vi "Create Tree.vi"(7 "Tree Refnum":refnum<vi>, 8 "error in":errorcluster, 9 "Parent Tag":string, 10 "palette data 2":T5={"display name"="", "view format"=0, "palette width"=4, "items"=[], "256 color icon"=bytes[0], "B&W color icon"=bytes[0], "help information"={"help tag"="", "help file path"=path ""}, "palette description"="", "synchronize information"={"synchronize with directory"=FALSE, "synchronize directory path"=path ""}} {"view format" items=["Icons", "Text", "Icons and Text"]}, 11 "palette data 1":T5={"display name"="", "view format"=0, "palette width"=4, "items"=[], "256 color icon"=bytes[0], "B&W color icon"=bytes[0], "help information"={"help tag"="", "help file path"=path ""}, "palette description"="", "synchronize information"={"synchronize with directory"=FALSE, "synchronize directory path"=path ""}} {"view format" items=["Icons", "Text", "Icons and Text"]}) -> (0 "error out":errorcluster, 2 "data array 2":cluster{"Label":string, "Data":variant}[](array[cluster]), 3 "data array 1":cluster{"Label":string, "Data":variant}[](array[cluster]))   [LabVIEW 2017]
uses:
  <vilib>/Palette API/Palette Menu/Public Type Define/View Format.ctl
  <vilib>/Palette API/Palette Menu/Public Type Define/Items.ctl
  <vilib>/Palette API/Palette Menu/Public Type Define/Item.ctl
  <vilib>/Palette API/Palette Menu/Public Type Define/Synchronize Info.ctl
  <vilib>/Palette API/Palette Menu/Palette Menu.lvlib
panel:
  in  "array size 1":i32
  in  "array size 2":i32
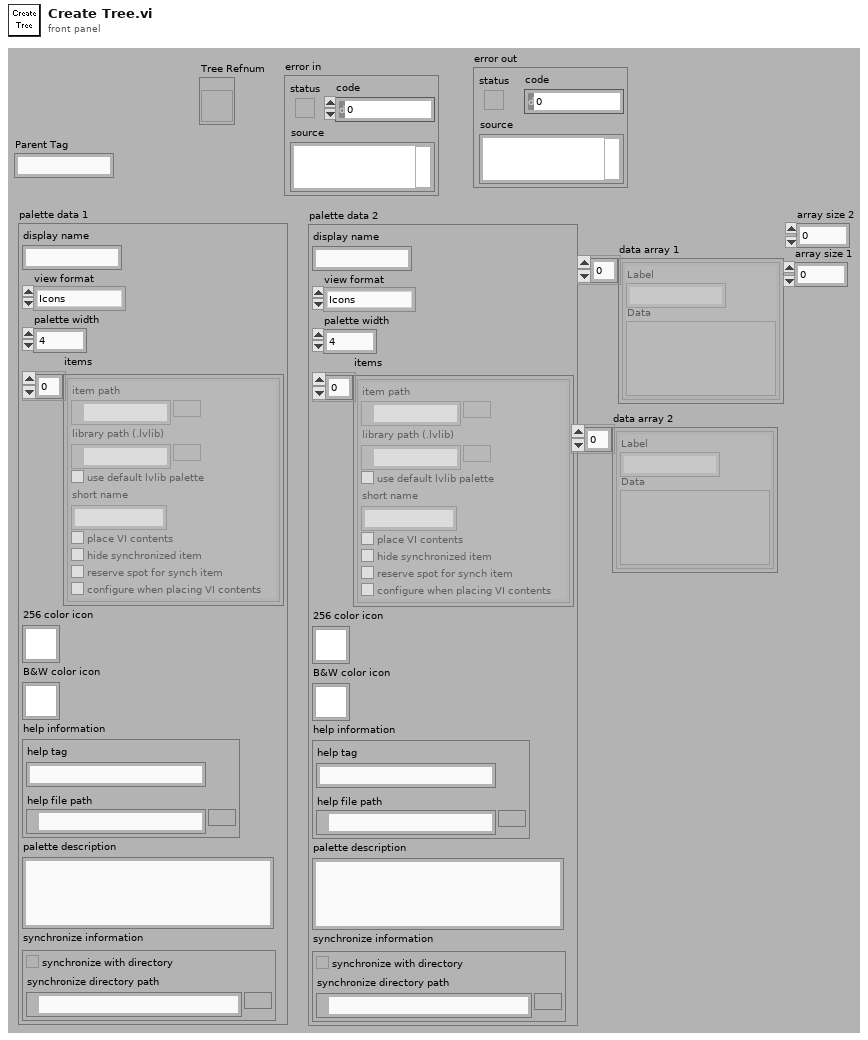
[diagram p1: front panel]
types:
  T1 = typedef "Palette Menu.lvlib/View Format.ctl" = u16
  T2 = typedef "Palette Menu.lvlib/Items.ctl" = T3[]
  T3 = typedef "Palette Menu.lvlib/Item.ctl" = cluster{"item path":path, "library path (.lvlib)":path, "use default lvlib palette":bool, "short name":string, "place VI contents":bool, "hide synchronized item":bool, "reserve spot for synch item":bool, "configure when placing VI contents":bool}
  T4 = typedef "Palette Menu.lvlib/Synchronize Info.ctl" = cluster{"synchronize with directory":bool, "synchronize directory path":path}
  T5 = cluster{"display name":string, "view format":T1, "palette width":i16, "items":T2, "256 color icon":picture, "B&W color icon":picture, "help information":cluster{"help tag":string, "help file path":path}, "palette description":string, "synchronize information":T4}
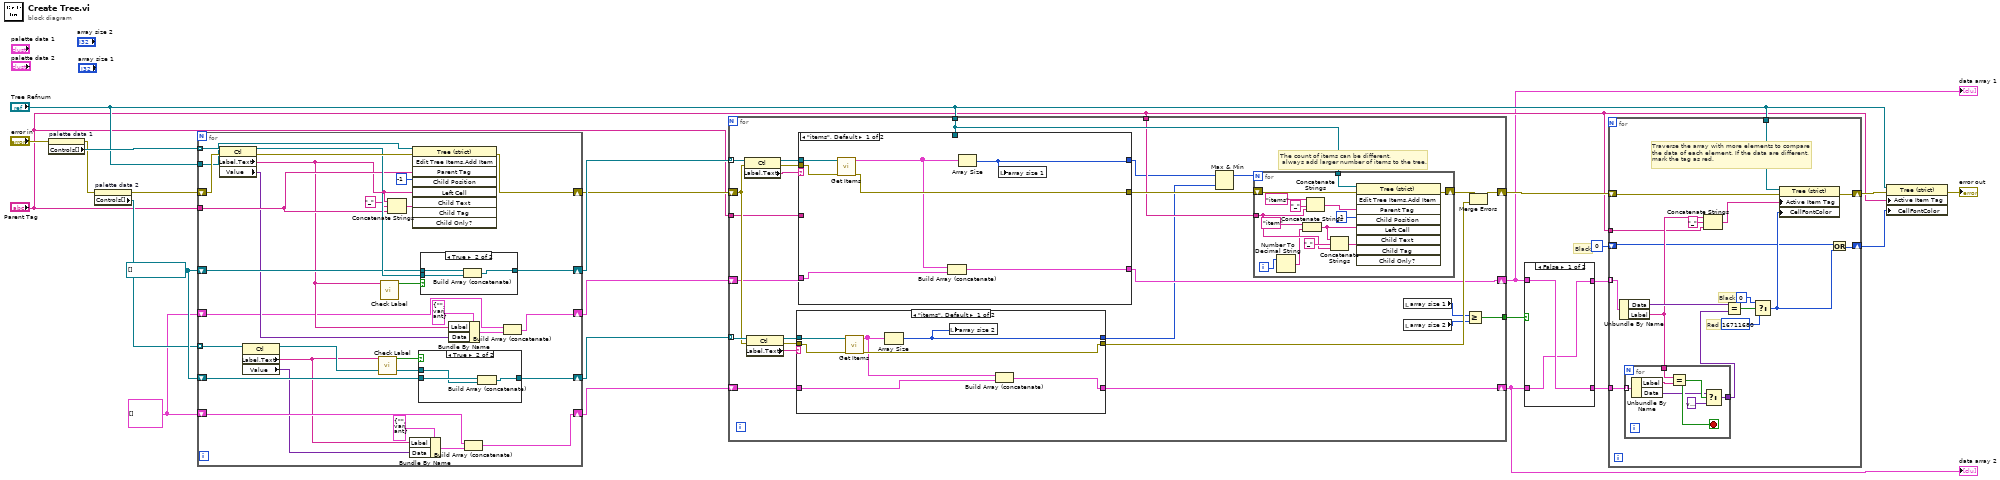
[diagram p0: block diagram]
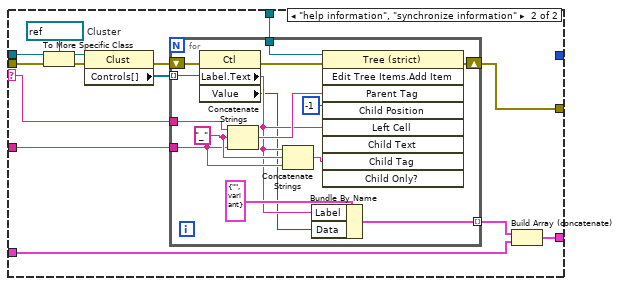
[diagram p3: hidden frame]
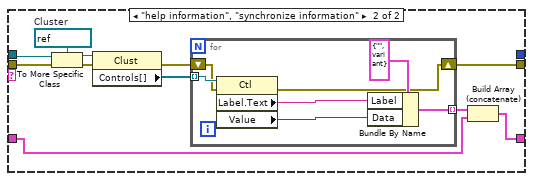
[diagram p4: hidden frame]
diagram:
  w16 = cluster{"Label":string, "Data":variant}[] []
  w24 = refnum<vi>[] []
  # "Black"
  n1 = property on="palette data 1" class="Clust (strict)"(error in="error in") -> (error out=w19:errorcluster, "Controls[]"=w21:refnum<vi>[])  [unwired: 1 in, 1 out]
  n2 = property on="palette data 2" class="Clust (strict)"(error in=w19) -> (error out=w18:errorcluster, "Controls[]"=w17:refnum<vi>[])  [unwired: 1 in, 1 out]
  n3 = for {
    tunnel: w21 -> [w53] mode=indexing
    shift-right: [w50] -> w22
    shift-left: w24 -> [w46]
    shift-right: [w37] -> w12
    shift-left: w18 -> [w49]
    tunnel: "Parent Tag" -> [w39]
    tunnel: w17 -> [w48] mode=indexing
    shift-right: [w45] -> w23
    shift-left: w24 -> [w44]
    tunnel: "Tree Refnum" -> [w43]
    shift-right: [w25] -> w15
    shift-left: w16 -> [w28]
    shift-right: [w31] -> w14
    shift-left: w16 -> [w32]
    n4 = property class="Ctl"(reference=w53, error in=w49) -> (reference out=w51:refnum<vi>, error out=w54:errorcluster, "Label.Text"=w33:string, "Value"=w34:variant)
    n5 = property class="Ctl"(reference=w48) -> (reference out=w47:refnum<vi>, "Label.Text"=w26:string, "Value"=w27:variant)  [unwired: 1 in, 1 out]
    n6 = call "Check Label.vi"("Label"=w26) -> ("Boolean"=w38:bool)  [unwired: 10 out]
    n7 = call "Check Label.vi"("Label"=w33) -> ("Boolean"=w52:bool)  [unwired: 10 out]
    n8 = Concatenate Strings(w33, "_" ("string"), w39) -> (w40:string)
    n9 = Bundle By Name(cluster=cluster{"Label":string, "Data":variant} {"Label"="", "Data"=variant} ("data cluster"), "Label"=w26, "Data"=w27) -> (w29:cluster{"Label":string, "Data":variant})
    n10 = invoke on="Invoke Node" class="Tree (strict)" method="Edit Tree Items.Add Item"(reference=w43, error in=w54, "Parent Tag"=w39, "Child Position"=-1, "Left Cell"=w33, "Child Tag"=w40) -> (error out=w37:errorcluster)  [unwired: 3 in, 8 out]
    n11 = case shown="True" w38 {
      tunnel: w47 -> [_ w56]
      tunnel: [w55 w58] -> w45
      tunnel: w44 -> [w55 w57]
      frame False {
      }
      frame True {
        n12 = Build Array (concatenate)(w57, w56) -> (w58:refnum<vi>[])
      }
    }
    n13 = case shown="True" w52 {
      tunnel: w51 -> [_ w60]
      tunnel: [w59 w62] -> w50
      tunnel: w46 -> [w59 w61]
      frame False {
      }
      frame True {
        n14 = Build Array (concatenate)(w61, w60) -> (w62:refnum<vi>[])
      }
    }
    n15 = Bundle By Name(cluster=cluster{"Label":string, "Data":variant} {"Label"="", "Data"=variant} ("data cluster"), "Label"=w33, "Data"=w34) -> (w35:cluster{"Label":string, "Data":variant})
    n16 = Build Array (concatenate)(w28, w29) -> (w25:cluster{"Label":string, "Data":variant}[])
    n17 = Build Array (concatenate)(w32, w35) -> (w31:cluster{"Label":string, "Data":variant}[])
  }
  n18 = for {
    tunnel: w22 -> [w88] mode=indexing
    shift-right: [w78] -> w13
    shift-left: w12 -> [w80]
    tunnel: w23 -> [w84] mode=indexing
    tunnel: "Tree Refnum" -> [w70]
    tunnel: "Parent Tag" -> [w77]
    shift-right: [w74] -> w1
    shift-left: w15 -> [w76]
    shift-right: [w73] -> w2
    shift-left: w14 -> [w75]
    tunnel: "Parent Tag" -> [w69]
    tunnel: [w67] -> w5
    # "The count of items can be different,\n always add larger number of items to the tree."
    n19 = property class="Ctl"(reference=w88, error in=w80) -> (reference out=w86:refnum<vi>, error out=w85:errorcluster, "Label.Text"=w87:string)
    n20 = property class="Ctl"(reference=w84, error in=w80) -> (reference out=w82:refnum<vi>, error out=w81:errorcluster, "Label.Text"=w83:string)
    n21 = case shown="\"items\", Default" w83 {
      tunnel: w82 -> [w145 w156]
      tunnel: w81 -> [w142 w155]
      tunnel: [w141 w146] -> w79
      tunnel: w76 -> [w144 w148]
      tunnel: [w143 w147] -> w74
      tunnel: [w139 _] -> w65
      frame "items", Default {
        n22 = call "Get Items.vi"("error in"=w142, "Ctl Refnum"=w145) -> ("error out"=w141:errorcluster, "items array"=w140:cluster{"Label":string, "Data":variant}[])  [unwired: 8 out]
        n23 = Array Size(array=w140) -> (size(s)=w139:i32)
        n24 = local write "array size 2"(w139) -> ()
        n25 = Build Array (concatenate)(w140, w144) -> (w143:cluster{"Label":string, "Data":variant}[])
      }
      frame "help information", "synchronize information" {
        w154 = refnum<vi> refnum  # Cluster
        n26 = To More Specific Class(target class=w154, reference=w156, error in=w155) -> (specific class reference=w152:refnum<vi>, error out=w153:errorcluster)
        n27 = property class="Clust"(reference=w152, error in=w153) -> (error out=w150:errorcluster, "Controls[]"=w151:refnum<vi>[])  [unwired: 1 out]
        n28 = for {
          tunnel: w151 -> [w163] mode=indexing
          shift-right: [w157] -> w146
          shift-left: w150 -> [w162]
          tunnel: [w158] -> w149 mode=indexing
          n29 = property class="Ctl"(reference=w163, error in=w162) -> (error out=w157:errorcluster, "Label.Text"=w160:string, "Value"=w159:variant)  [unwired: 1 out]
          n30 = Bundle By Name(cluster=cluster{"Label":string, "Data":variant} {"Label"="", "Data"=variant} ("data cluster"), "Label"=w160, "Data"=w159) -> (w158:cluster{"Label":string, "Data":variant})
        }
        n31 = Build Array (concatenate)(w149, w148) -> (w147:cluster{"Label":string, "Data":variant}[])
      }
    }
    n32 = case shown="\"items\", Default" w87 {
      selector: w87 -> [_ w118]
      tunnel: w86 -> [w109 w123]
      tunnel: w85 -> [w106 w122]
      tunnel: [w105 w116] -> w72
      tunnel: w77 -> [_ w114]
      tunnel: w75 -> [w108 w112]
      tunnel: [w107 w111] -> w73
      tunnel: w70 -> [_ w110]
      tunnel: [w103 _] -> w66
      frame "items", Default {
        n33 = call "Get Items.vi"("error in"=w106, "Ctl Refnum"=w109) -> ("error out"=w105:errorcluster, "items array"=w104:cluster{"Label":string, "Data":variant}[])  [unwired: 8 out]
        n34 = Build Array (concatenate)(w104, w108) -> (w107:cluster{"Label":string, "Data":variant}[])
        n35 = Array Size(array=w104) -> (size(s)=w103:i32)
        n36 = local write "array size 1"(w103) -> ()
      }
      frame "help information", "synchronize information" {
        w121 = refnum<vi> refnum  # Cluster
        n37 = To More Specific Class(target class=w121, reference=w123, error in=w122) -> (specific class reference=w119:refnum<vi>, error out=w120:errorcluster)
        n38 = property class="Clust"(reference=w119, error in=w120) -> (error out=w117:errorcluster, "Controls[]"=w115:refnum<vi>[])  [unwired: 1 out]
        n39 = for {
          tunnel: w115 -> [w138] mode=indexing
          tunnel: w118 -> [w132]
          shift-right: [w135] -> w116
          shift-left: w117 -> [w134]
          tunnel: w110 -> [w133]
          tunnel: w114 -> [w129]
          tunnel: [w124] -> w113 mode=indexing
          w130 = "_" ("string")
          n40 = property class="Ctl"(reference=w138, error in=w134) -> (error out=w137:errorcluster, "Label.Text"=w126:string, "Value"=w125:variant)  [unwired: 1 out]
          n41 = Concatenate Strings(w132, w130, w129) -> (w131:string)
          n42 = Concatenate Strings(w126, w130, w129) -> (w128:string)
          n43 = Bundle By Name(cluster=cluster{"Label":string, "Data":variant} {"Label"="", "Data"=variant} ("data cluster"), "Label"=w126, "Data"=w125) -> (w124:cluster{"Label":string, "Data":variant})
          n44 = invoke on="Invoke Node" class="Tree (strict)" method="Edit Tree Items.Add Item"(reference=w133, error in=w137, "Parent Tag"=w131, "Child Position"=-1, "Left Cell"=w126, "Child Tag"=w128) -> (error out=w135:errorcluster)  [unwired: 3 in, 8 out]
        }
        n45 = Build Array (concatenate)(w113, w112) -> (w111:cluster{"Label":string, "Data":variant}[])
      }
    }
    n46 = Max & Min(x=w66, y=w65) -> (max(x,y)=w68:i32)  [unwired: 1 out]
    n47 = for {
      N: w68 -> [_]
      tunnel: w70 -> [w101]
      shift-right: [w100] -> w71
      shift-left: w72 -> [w99]
      tunnel: w69 -> [w95]
      i -> [w90]
      n48 = Number To Decimal String(number=w90) -> (decimal integer string=w92:string)  [unwired: 1 out]
      n49 = Concatenate Strings("item" ("string"), w92) -> (w91:string)
      n50 = Concatenate Strings("items" ("Parent Tag"), "_" ("string"), w95) -> (w97:string)
      n51 = Concatenate Strings(w91, "_" ("string"), w95) -> (w94:string)
      n52 = invoke on="Invoke Node" class="Tree (strict)" method="Edit Tree Items.Add Item"(reference=w101, error in=w99, "Parent Tag"=w97, "Child Position"=-1, "Left Cell"=w91, "Child Tag"=w94) -> (error out=w100:errorcluster)  [unwired: 3 in, 8 out]
    }
    n53 = local read "array size 1"() -> (w64:i32)
    n54 = local read "array size 2"() -> (w63:i32)
    n55 = Greater Or Equal?(x=w64, y=w63) -> (x >= y?=w67:bool)
    n56 = Merge Errors(w71, w79) -> (w78:errorcluster)
  }
  "data array 1" <- w2
  "data array 2" <- w1
  n57 = case shown="False" w5 {
    tunnel: [w164 w167] -> w4
    tunnel: w2 -> [w165 w167]
    tunnel: w1 -> [w164 w166]
    tunnel: [w165 w166] -> w3
    frame False {
    }
    frame True {
    }
  }
  n58 = for {
    shift-right: [w176] -> w10
    shift-left: w13 -> [w177]
    tunnel: w4 -> [w184] mode=indexing
    tunnel: w3 -> [w171]
    tunnel: "Tree Refnum" -> [w178]
    tunnel: "Parent Tag" -> [w173]
    shift-right: [w169] -> w7
    shift-left: u32 0 -> [w168]
    # "Traverse the array with more elements to compare\nthe data of each element. If the data are different, \nmark the tag as red."
    # "Red"
    # "Black"
    n59 = Unbundle By Name(w184) -> ("Data"=w181:variant, "Label"=w175:string)
    n60 = for {
      tunnel: w171 -> [w191] mode=indexing
      tunnel: w175 -> [w189]
      tunnel: [w185] -> w180
      stop <- w188 stop-if-true
      n61 = Unbundle By Name(w191) -> ("Label"=w190:string, "Data"=w187:variant)
      n62 = Equal?(x=w189, y=w190) -> (x = y?=w188:bool)
      n63 = Select(t=w187, s=w188, f=variant) -> (s? t:f=w185:variant)
    }
    n64 = Concatenate Strings(w175, "_" ("string"), w173) -> (w172:string)
    n65 = Equal?(x=w181, y=w180) -> (x = y?=w183:bool)
    n66 = Select(t=u32 0, s=w183, f=u32 16711680) -> (s? t:f=w170:u32)
    n67 = property class="Tree (strict)"(reference=w178, error in=w177, "Active Item Tag"=w172, "CellFontColor"=w170) -> (error out=w176:errorcluster)  [unwired: 1 out]
    n68 = Or(x=w168, y=w170) -> (x .or. y?=w169:u32)
  }
  n69 = property class="Tree (strict)"(reference="Tree Refnum", error in=w10, "Active Item Tag"="Parent Tag", "CellFontColor"=w7) -> (error out=→"error out":errorcluster)  [unwired: 1 out]
